vi "Create Array.vi"(8 "error in (no error)":errorcluster, 10 "Default Type (if empty)":variant, 11 "Elements":variant[](array[variant])) -> (0 "error out":errorcluster, 3 "Array":variant)   [LabVIEW 2019, in "labview_json.lvlib"]
uses:
  labview_json.lvlib
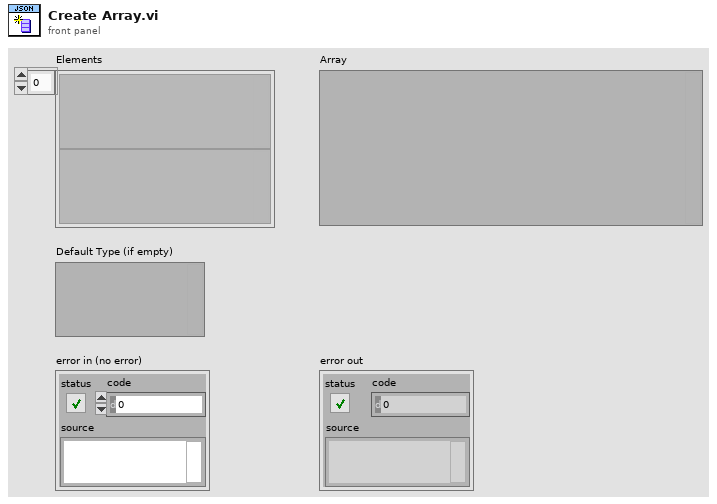
[diagram p1: front panel]
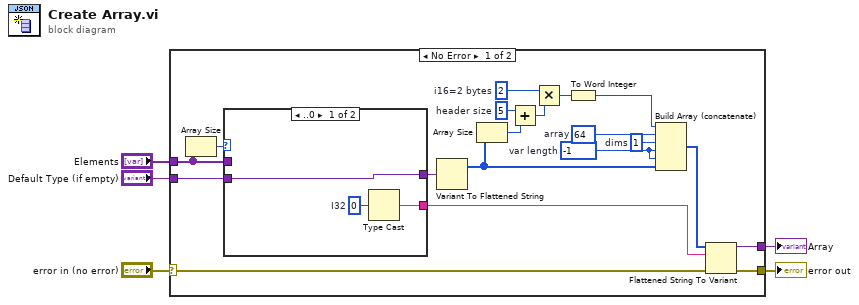
[diagram p0: block diagram]
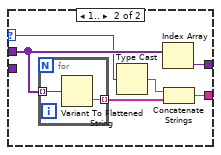
[diagram p2: hidden frame]
diagram:
  n1 = case shown="No Error" "error in (no error)" {
    selector: "error in (no error)" -> [w22 w36]
    tunnel: "Elements" -> [w23 _]
    tunnel: [w21 w36] -> w3
    tunnel: [w20 _] -> w2
    tunnel: "Default Type (if empty)" -> [w6 _]
    frame No Error {
      w9 = i16 -1  # var length
      w10 = i16 1  # dims
      w13 = i16 64  # array
      w17 = 2  # i16=2 bytes
      w18 = 5  # header size
      n2 = Array Size(array=w23) -> (size(s)=w24:i32)
      n3 = case shown="..0" w24 {
        selector: w24 -> [_ w28]
        tunnel: w23 -> [_ w33]
        tunnel: [w26 w30] -> w12
        tunnel: [w25 w29] -> w7
        tunnel: w6 -> [w25 _]
        frame ..0 {
          w27 = 0  # I32
          n4 = Type Cast(x=w27) -> (*(type *) &x=w26:string)  [unwired: 1 in]
        }
        frame 1.. {
          n5 = for {
            tunnel: w33 -> [w35] mode=indexing
            tunnel: [w34] -> w32 mode=indexing
            n6 = Variant To Flattened String(Variant=w35) -> (data string=w34:string)  [unwired: 1 out]
          }
          n7 = Type Cast(x=w28) -> (*(type *) &x=w31:string)  [unwired: 1 in]
          n8 = Index Array(array=w33) -> (element=w29:variant)  [unwired: 1 in]
          n9 = Concatenate Strings(w31, w32) -> (w30:string)
        }
      }
      n10 = Variant To Flattened String(Variant=w7) -> (1:w8:i16[])  [unwired: 1 out]
      n11 = Array Size(array=w8) -> (size(s)=w11:i32)
      n12 = Add(x=w18, y=w11) -> (x+y=w16:i32)
      n13 = Multiply(x=w17, y=w16) -> (x*y=w15:i32)
      n14 = To Word Integer(number=w15) -> (16bit integer=w14:i16)
      n15 = Build Array (concatenate)(w14, w13, w10, w9, w9, w8) -> (w19:i16[])
      n16 = Flattened String To Variant(4:w22, 6:w12, 7:w19) -> (0:w21:errorcluster, 3:w20:variant)
    }
    frame Error {
    }
  }
  "error out" <- w3
  "Array" <- w2
